vi "libdaq_pwm_set.vi"(0 "error in (no error)":errorcluster, 1 "device_name":string, 2 "module_name":string, 3 "period":i32, 4 "pulse":i32, 5 "count":i32) -> (14 "error out":errorcluster, 15 "device_name":string, 16 "module_name":string)   [LabVIEW 2010, in "libdaqVI.lvlib"]
uses:
  libdaqVI.lvlib
  dll/daqlib.dll
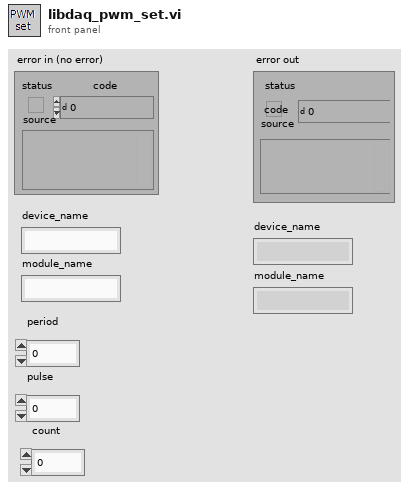
[diagram p1: front panel]
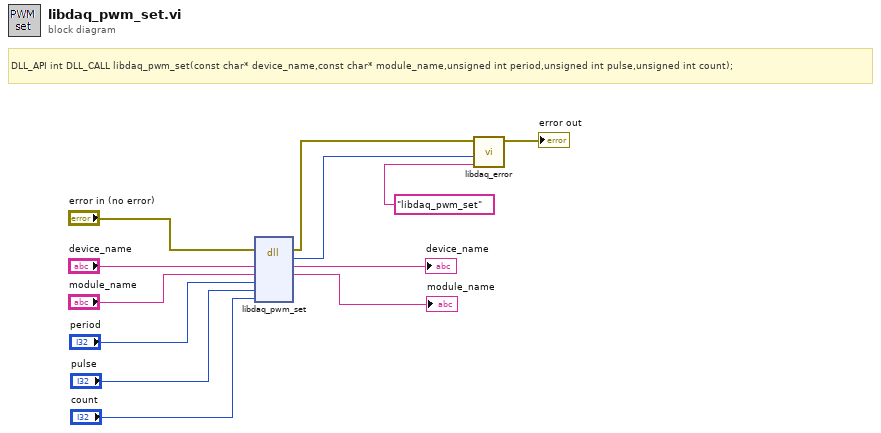
[diagram p0: block diagram]
diagram:
  # "DLL_API int DLL_CALL libdaq_pwm_set(const char* device_name,const char* module_name,unsigned int period,unsigned int pulse,unsigned int count);"
  n1 = dll-call lib="E:/Product/Example/DAQ-USB3212/Labview/labview_2010/libdaqVI/dll/daqlib.dll" fn="libdaq_pwm_set"(error in="error in (no error)", "device_name"="device_name", "module_name"="module_name", "period"="period", "pulse"="pulse", "count"="count") -> (error out=w7:errorcluster, "return type"=w5:i32, "device_name"=→"device_name":string, "module_name"=→"module_name":string)  [unwired: 5 in, 1 out]
  n2 = call "libdaq_error.vi"("error source"="libdaq_pwm_set", "error code"=w5, "错误输入（无错误）"=w7) -> ("错误输出"=→"error out":errorcluster)  [unwired: 8 in]
